vi "Close Serial Driver.vi"(1 "port number":i32) -> (0 "error":i32)   [LabVIEW 2020]
doc: "Closes the specified port."
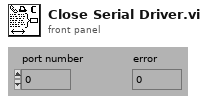
[diagram p1: front panel]
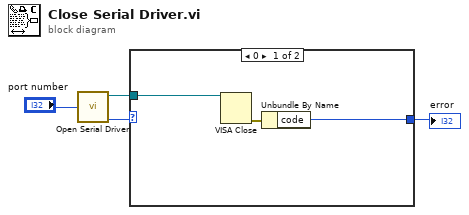
[diagram p0: block diagram]
diagram:
  n1 = call "Open Serial Driver.vi"("port number"="port number") -> ("input refnum"=w2:refnum<visa-resource-name>, "output error"=w3:i32)  [unwired: 2 out]
  n2 = case shown="0" w3 {
    selector: w3 -> [_ w8]
    tunnel: w2 -> [w7 _]
    tunnel: [w5 w8] -> w1
    frame 0 {
      n3 = VISA Close(VISA resource name=w7) -> (error out=w6:errorcluster)  [unwired: 1 in]
      n4 = Unbundle By Name(w6) -> ("code"=w5:i32)
    }
    frame 1, Default {
    }
  }
  "error" <- w1
